vi "EMB_Debug_Map_RV_ResolveSymbols.vi"(8 "error in (no error)":errorcluster, 10 "Target":string, 11 "VI Name":string) -> (0 "error out":errorcluster)   [LabVIEW 2011]
uses:
  <vilib>/LabVIEW Targets/Embedded/Debug/DD/utils/EMB_Debug_DD_GetSetAttrib_String.vi
panel:
  out "Sub VI Name":string
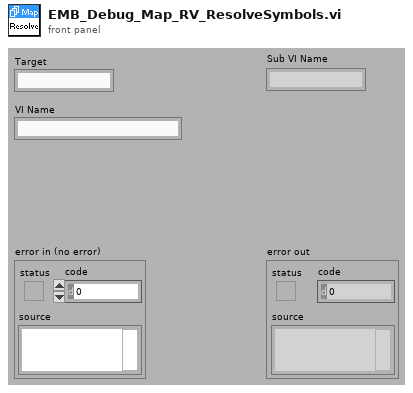
[diagram p1: front panel]
types:
  T1 = enum16{"UV_STATUS_SUCCESS", "UV_STATUS_FAILED", "UV_STATUS_NO_PROJECT", "UV_STATUS_WRITE_PROTECTED", "UV_STATUS_NO_TARGET", "UV_STATUS_NO_TOOLSET", "UV_STATUS_TARGET_BLOCKED", "UV_STATUS_ALREADY_PRESENT", "UV_STATUS_INVALID_NAME", "UV_STATUS_NOT_FOUND", "UV_STATUS_WRONG_MODE", "UV_STATUS_TARGET_EXECUTING", "UV_STATUS_TARGET_STOPPED", "UV_STATUS_PARSE_ERROR", "UV_STATUS_OUT_OF_RANGE"}
  T2 = typedef "EMB_Debug_DD_MemType.ctl" = enum16{"Signal", "Control"}
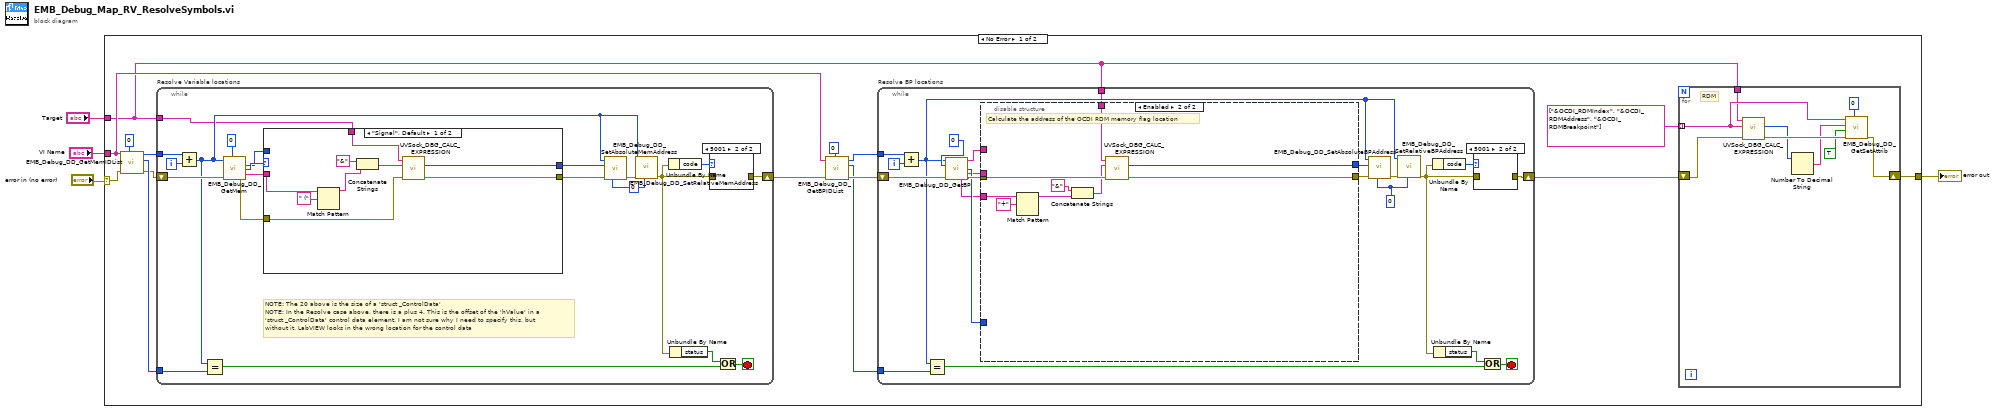
[diagram p0: block diagram]
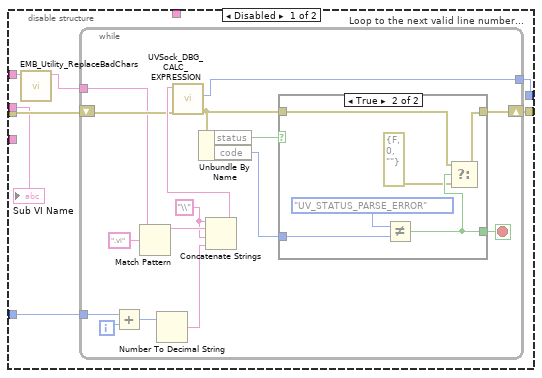
[diagram p2: hidden frame]
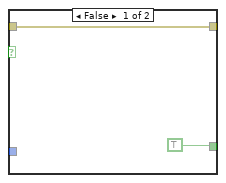
[diagram p3: hidden frame]
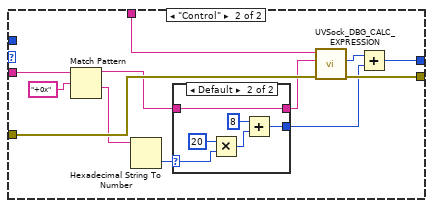
[diagram p5: hidden frame]
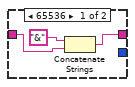
[diagram p6: hidden frame]
diagram:
  n1 = case shown="No Error" "error in (no error)" {
    selector: "error in (no error)" -> [w15 w144]
    tunnel: [w6 w144] -> w3
    tunnel: "VI Name" -> [w14 _]
    tunnel: "Target" -> [w5 _]
    frame No Error {
      n2 = call <vilib>:"EMB_Debug_DD_GetMemIDList.vi"("target ID"=u32 0, "error in (no error)"=w15, "VI Name"=w14) -> ("error out"=w16:errorcluster, "End ID"=w17:u32, "Start ID"=w18:u32)  [unwired: 6 out]
      n3 = while "Resolve Variable locations" {
        tunnel: w18 -> [w92]
        tunnel: w17 -> [w111]
        shift-right: [w103] -> w11
        shift-left: w16 -> [w109]
        tunnel: w5 -> [w94]
        i -> [w112]
        stop <- w108 stop-if-true
        w99 = u32 0 ("target ID")
        # "NOTE: The 20 above is the size of a 'struct _ControlData'\nNOTE: In the Resolve case above, there is a plus 4. This is the offset of the 'hValue' in a  \n'struct _ControlData' control data element. I am not sure why I need to specify this, but \nwithout it, LabVIEW looks in the wrong location for the control data"
        n4 = Add(x=w92, y=w112) -> (x+y=w100:u32)
        n5 = Equal?(x=w100, y=w111) -> (x = y?=w106:bool)
        n6 = call <vilib>:"EMB_Debug_DD_GetMem.vi"("target ID"=u32 0, "error in (no error)"=w109, "Memory ID"=w100) -> ("error out"=w96:errorcluster, "Memory Type"=w98:T2, "Signal/Control ID"=w93:u32, "Relative Address"=w102:string)  [unwired: 5 out]
        n7 = case shown="\"Signal\", Default" w98 {
          tunnel: w102 -> [w120 w133]
          tunnel: [w117 w127] -> w97
          tunnel: w96 -> [w116 w131]
          tunnel: [w115 w130] -> w95
          tunnel: w94 -> [w113 w126]
          tunnel: w93 -> [_ _]
          frame "Signal", Default {
            n8 = Match Pattern(string=w120, regular expression=" (") -> (before substring=w118:string)  [unwired: 4 out]
            n9 = Concatenate Strings("&" ("string"), w118) -> (w114:string)
            n10 = call "UVSock_DBG_CALC_EXPRESSION.vi"("error in (no error)"=w116, "Expression"=w114, "Target"=w113) -> ("error out"=w115:errorcluster, "Value"=w117:u64)  [unwired: 7 out]
          }
          frame "Control" {
            n11 = Match Pattern(string=w133, regular expression="+0x") -> (before substring=w123:string, after substring=w129:string)  [unwired: 3 out]
            n12 = Hexadecimal String To Number(string=w129) -> (number=w124:u32)  [unwired: 3 out]
            n13 = case shown="Default" w124 {
              selector: w124 -> [_ w138]
              tunnel: [_ w140] -> w128
              tunnel: w123 -> [w136 w137]
              tunnel: [w134 w137] -> w122
              frame 65536 {
                n14 = Concatenate Strings("&" ("string"), w136) -> (w134:string)
              }
              frame Default {
                n15 = Multiply(x=u32 20, y=w138) -> (x*y=w141:u32)
                n16 = Add(x=u64 8, y=w141) -> (x+y=w140:u64)
              }
            }
            n17 = call "UVSock_DBG_CALC_EXPRESSION.vi"("error in (no error)"=w131, "Expression"=w122, "Target"=w126) -> ("error out"=w130:errorcluster, "Value"=w125:u64)  [unwired: 7 out]
            n18 = Add(x=w125, y=w128) -> (x+y=w127:u64)
          }
        }
        n19 = call <vilib>:"EMB_Debug_DD_SetAbsoluteMemAddress.vi"("target ID"=w99, "error in (no error)"=w95, "Address"=w97, "Memory ID"=w100) -> ("error out"=w101:errorcluster)  [unwired: 7 out]
        n20 = call <vilib>:"EMB_Debug_DD_SetRelativeMemAddress.vi"("target ID"=w99, "error in (no error)"=w101, "Memory ID"=w100) -> ("error out"=w104:errorcluster)  [unwired: 1 in, 7 out]
        n21 = Unbundle By Name(w104) -> ("code"=w105:i32)
        n22 = Unbundle By Name(w104) -> ("status"=w107:bool)
        n23 = case shown="5001" w105 {
          tunnel: w104 -> [w143 _]
          tunnel: [w143 _] -> w103
          frame 0, Default {
          }
          frame 5001 {
          }
        }
        n24 = Or(x=w107, y=w106) -> (x .or. y?=w108:bool)
      }
      n25 = call <vilib>:"EMB_Debug_DD_GetBPIDList.vi"("target ID"=u32 0, "error in (no error)"=w11, "VI Name"=w14) -> ("error out"=w12:errorcluster, "End ID"=w10:u32, "Start ID"=w9:u32)  [unwired: 6 out]
      n26 = while "Resolve BP locations" {
        tunnel: w9 -> [w50]
        tunnel: w10 -> [w48]
        shift-right: [w44] -> w8
        shift-left: w12 -> [w41]
        tunnel: w5 -> [w29]
        i -> [w49]
        stop <- w47 stop-if-true
        w34 = u32 0 ("target ID")
        n27 = Add(x=w50, y=w49) -> (x+y=w33:u32)
        n28 = Equal?(x=w33, y=w48) -> (x = y?=w45:bool)
        n29 = call <vilib>:"EMB_Debug_DD_GetBP.vi"("Breakpoint ID"=w33, "target ID"=u32 0, "error in (no error)"=w41) -> ("VI Name"=w38:string, "Breakpoint Line"=w39:u32, "Sub VI Name"=w37:string, "Breakpoint Relative Address"=w30:string, "error out"=w40:errorcluster)  [unwired: 8 out]
        n30 = disable-structure shown="Enabled" {
          disable-tunnel: w40 -> [w57 w86]
          disable-tunnel: w39 -> [w56 _]
          disable-tunnel: w38 -> [w55 _]
          disable-tunnel: w37 -> [w53 _]
          disable-tunnel: [w52 w84] -> w36
          disable-tunnel: [w51 w85] -> w35
          disable-tunnel: w30 -> [_ w90]
          disable-tunnel: w29 -> [_ w83]
          frame Disabled {
            n31 = call <vilib>:"EMB_Utility_ReplaceBadChars.vi"("Input String"=w55) -> ("Output String"=w54:string)  [unwired: 10 in]
            n32 = while "Loop to the next valid line number..." {
              tunnel: [w58] -> w51
              tunnel: w56 -> [w73]
              tunnel: w54 -> [w59]
              shift-right: [w60] -> w52
              shift-left: w57 -> [w62]
              i -> [w72]
              stop <- w63 stop-if-true
              w69 = "\\" ("string")
              n33 = Add(x=w73, y=w72) -> (x+y=w68:u32)
              n34 = Match Pattern(string=w59, regular expression=".vi") -> (before substring=w70:string)  [unwired: 1 in, 3 out]
              n35 = Number To Decimal String(number=w68) -> (decimal integer string=w67:string)  [unwired: 1 in]
              n36 = Concatenate Strings(w69, w70, w69, w67) -> (w66:string)
              n37 = call "UVSock_DBG_CALC_EXPRESSION.vi"("error in (no error)"=w62, "Target"=w66) -> ("error out"=w61:errorcluster, "Value"=w58:u64)  [unwired: 7 in, 1 out]
              n38 = Unbundle By Name(w61) -> ("status"=w65:bool, "code"=w64:i32)
              n39 = case shown="True" w65 {
                tunnel: w64 -> [_ w81]
                tunnel: [TRUE w78] -> w63
                tunnel: w61 -> [w74 w77]
                tunnel: [w74 w79] -> w60
                frame False {
                }
                frame True {
                  n40 = Not Equal?(x=T1."UV_STATUS_PARSE_ERROR", y=w81) -> (x != y?=w78:bool)
                  n41 = Select(t=w77, s=w78, f=errorcluster {"status"=FALSE, "code"=0, "source"=""}) -> (s? t:f=w79:errorcluster)
                }
              }
            }
            "Sub VI Name" <- w53
          }
          frame Enabled {
            # "Calculate the address of the OCDI RDM memory flag location"
            n42 = Match Pattern(string=w90, regular expression="+") -> (before substring=w87:string)  [unwired: 4 out]
            n43 = Concatenate Strings("&" ("string"), w87) -> (w82:string)
            n44 = call "UVSock_DBG_CALC_EXPRESSION.vi"("error in (no error)"=w86, "Expression"=w82, "Target"=w83) -> ("error out"=w84:errorcluster, "Value"=w85:u64)  [unwired: 7 out]
          }
        }
        n45 = call <vilib>:"EMB_Debug_DD_SetAbsoluteBPAddress.vi"("target ID"=w34, "error in (no error)"=w36, "Breakpoint Address"=w35, "Breakpoint ID"=w33) -> ("error out"=w32:errorcluster)  [unwired: 7 out]
        n46 = call <vilib>:"EMB_Debug_DD_SetRelativeBPAddress.vi"("target ID"=w34, "error in (no error)"=w32, "Breakpoint ID"=w33) -> ("error out"=w31:errorcluster)  [unwired: 1 in, 7 out]
        n47 = Unbundle By Name(w31) -> ("code"=w43:i32)
        n48 = Unbundle By Name(w31) -> ("status"=w46:bool)
        n49 = case shown="5001" w43 {
          tunnel: w31 -> [w91 _]
          tunnel: [w91 _] -> w44
          frame 0, Default {
          }
          frame 5001 {
          }
        }
        n50 = Or(x=w46, y=w45) -> (x .or. y?=w47:bool)
      }
      n51 = for {
        tunnel: string[] ["&OCDI_RDMIndex", "&OCDI_RDMAddress", "&OCDI_RDMBreakpoint"] -> [w21] mode=indexing
        shift-right: [w22] -> w6
        shift-left: w8 -> [w28]
        tunnel: w5 -> [w20]
        # "RDM"
        n52 = call "UVSock_DBG_CALC_EXPRESSION.vi"("error in (no error)"=w28, "Expression"=w21, "Target"=w20) -> ("error out"=w27:errorcluster, "Value"=w25:u64)  [unwired: 7 out]
        n53 = Number To Decimal String(number=w25) -> (decimal integer string=w24:string)  [unwired: 1 out]
        n54 = call-poly <vilib>:"EMB_Debug_DD_GetSetAttrib.vi"("target ID"=u32 0, "error in (no error)"=w27, "set"=TRUE, "value"=w24, "name"=w21) -> ("error out"=w22:errorcluster)  [unwired: 6 out]
      }
    }
    frame Error {
    }
  }
  "error out" <- w3
